vi "omni1.vi"   [LabVIEW 2012, in "Omni2013.lvrbt"]
uses:
  Omni2013.lvrbt
  <vilib>/NXT/Hardware/Plugins/Tetrix DC Motor/TetrixDCMotorAddress.ctl
  <vilib>/NXT/Hardware/Plugins/Tetrix 180 deg Servo/Tetrix180ServoAddress.ctl
  <vilib>/NXT/Dual Mode Library/Display/drawNumber_float.vi
  <vilib>/NXT/NXTIO Xnodes/NXTIONodeSubVIs/TETRIX IO Move DC Motors.vi
  <vilib>/NXT/NXTIO Xnodes/NXTIONodeSubVIs/TETRIX IO Move Servos.vi
  <vilib>/NXT/Dual Mode Library/Display/drawText_Center.vi
  <vilib>/NXT/NXTIO Xnodes/AddressXNode/NXTIOAddress.xnode
  <vilib>/NXT/NXTIO Xnodes/NXTIOXNode/NXTIO.xnode
  <vilib>/NXT/Subs/LVHSConnector.ctl
  <vilib>/NXT/LegoClasses/BrickReference/BrickReference.lvclass
panel:
  # "This VI was generated based on your configuration in the Remote Control Editor. You may modify the code as needed for your robot. To test this program for an FTC match, return to the Remote Control Editor, select the \"Run Program\" tab, and choose \"FTC Game\"."
types:
  T1 = typedef "TetrixDCMotorAddress.ctl" = i16
  T2 = cluster{"TetrixDCMotor":T1, "TetrixDCMotor 2":T1}
  T3 = typedef "LVHSConnector.ctl" = refnum<class "BrickReference.lvclass">
  T4 = typedef "FTC ControllerState.ctl" = cluster{"Left X":i8, "Left Y":i8, "Right X":i8, "Right Y":i8, "Button Encoding 9-12":u8, "Button Encoding 1-8":u8, "POV":T5}
  T5 = typedef "FTC POVState.ctl" = i8
  T6 = typedef "FTC ButtonEventType.ctl" = enum16{"Pressed", "Released"}
  T7 = cluster{"Button ID":enum16{"None", "Button 1", "Button 2", "Button 3", "Button 4", "Button 5", "Button 6", "Button 7", "Button 8", "Button 9", "Button 10", "Button 11", "Button 12", "POV Up", "POV Up Right", "POV Right", "POV Down Right", "POV Down", "POV Down Left", "POV Left", "POV Up Left"}, "Event Type":T6}[]
  T8 = enum16{"None", "Button 1", "Button 2", "Button 3", "Button 4", "Button 5", "Button 6", "Button 7", "Button 8", "Button 9", "Button 10", "Button 11", "Button 12", "POV Up", "POV Up Right", "POV Right", "POV Down Right", "POV Down", "POV Down Left", "POV Left", "POV Up Left"}
  T9 = typedef "Tetrix180ServoAddress.ctl" = i16
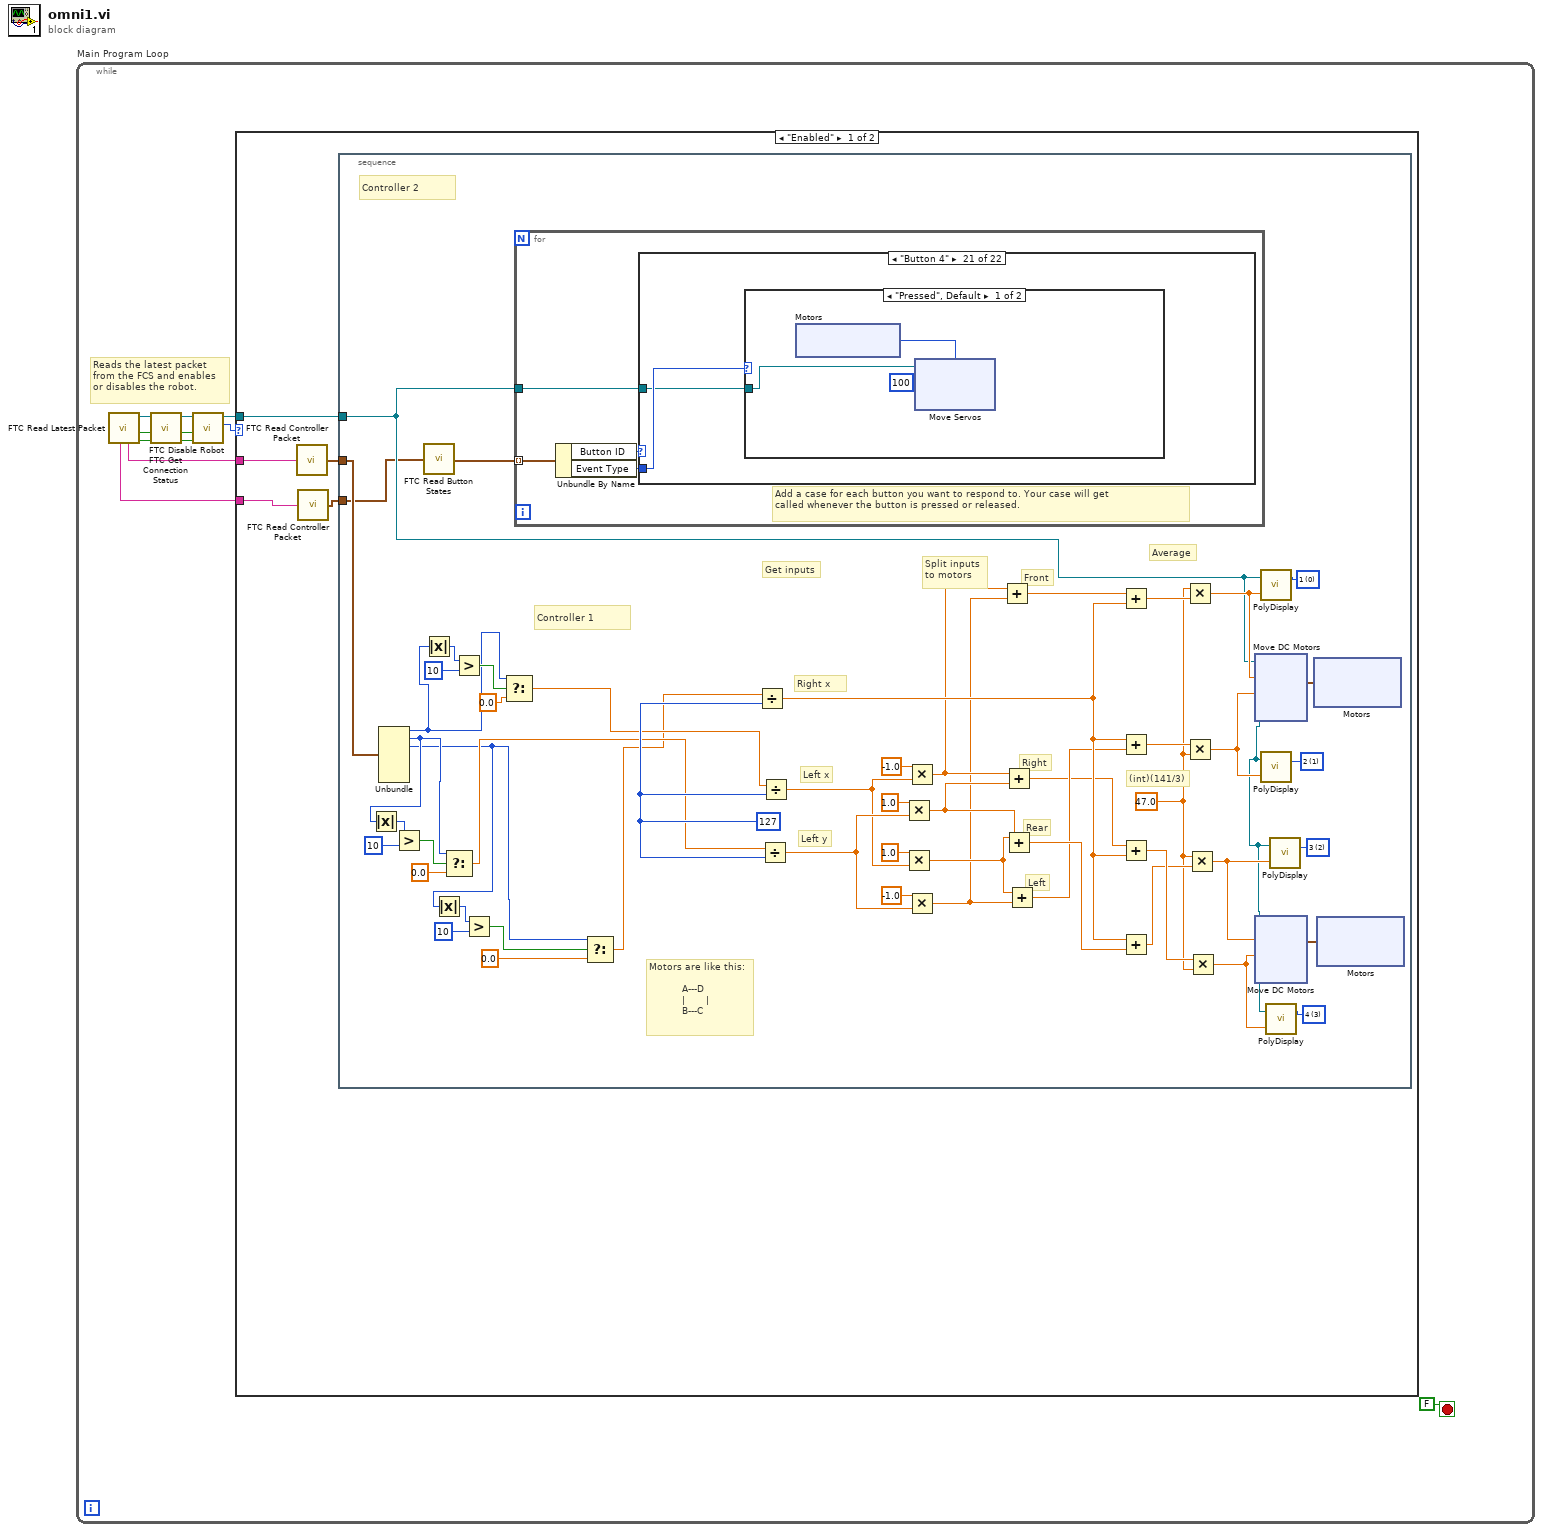
[diagram p0: block diagram]
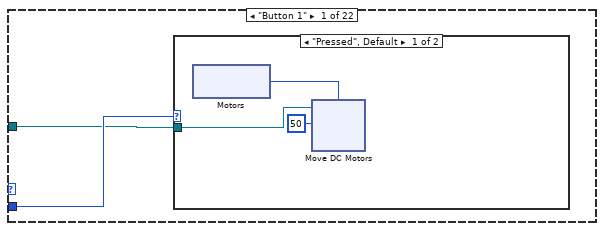
[diagram p2: hidden frame]
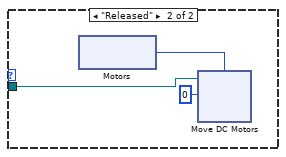
[diagram p3: hidden frame]
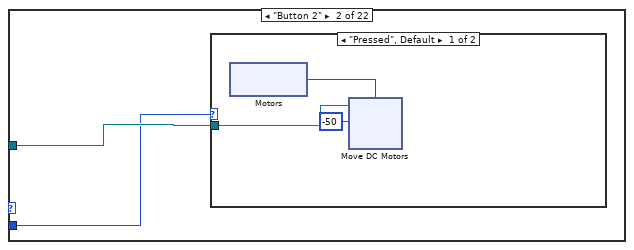
[diagram p4: hidden frame]
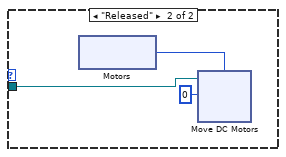
[diagram p5: hidden frame]
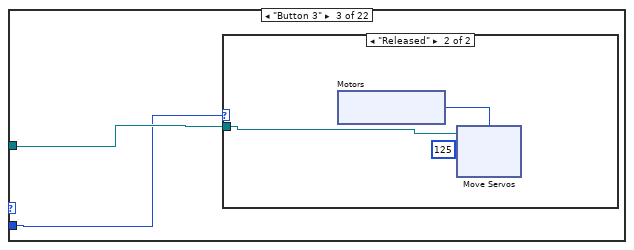
[diagram p6: hidden frame]
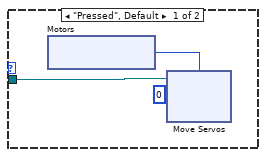
[diagram p7: hidden frame]
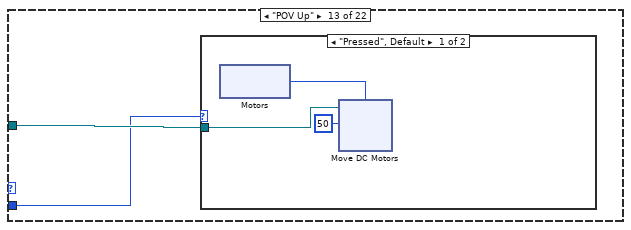
[diagram p17: hidden frame]
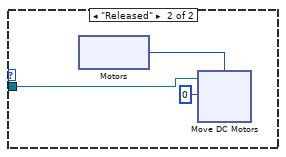
[diagram p18: hidden frame]
diagram:
  n1 = while "Main Program Loop" {
    stop <- FALSE stop-if-true
    # "Reads the latest packet\nfrom the FCS and enables\nor disables the robot."
    n2 = call <vilib>:"FTC Read Latest Packet.vi"() -> ("Packet Received?"=w9:bool, "Stopped?"=w6:bool, "NXT"=w8:T3, "Controller 1"=w10:string, "Controller 2"=w1:string)  [unwired: 6 in, 1 out]
    n3 = call <vilib>:"FTC Get Connection Status.vi"("Packet Received?"=w9, "Stopped?"=w6, "NXT"=w8) -> ("Online?"=w3:bool, "Stopped?"=w4:bool, "NXT"=w5:T3)  [unwired: 5 in]
    n4 = call <vilib>:"FTC Disable Robot.vi"("Online?"=w3, "Stopped?"=w4, "NXT"=w5) -> ("Enabled?"=w7:enum16{"Disabled", "Enabled"}, "NXT"=w2:T3)  [unwired: 3 in]
    n5 = case "disableCase" shown="\"Enabled\"" w7 {
      tunnel: w10 -> [w16 _]
      tunnel: w2 -> [w14 w249]
      tunnel: w1 -> [w13 _]
      frame "Enabled" {
        n6 = call <vilib>:"FTC Read Controller Packet.vi"("Packet"=w16) -> ("Controller State"=w15:T4)  [unwired: 4 in]
        n7 = call <vilib>:"FTC Read Controller Packet.vi"("Packet"=w13) -> ("Controller State"=w12:T4)  [unwired: 4 in]
        n8 = stacked-sequence "controller1Actions" {
          tunnel: w15 -> [w53]
          tunnel: w14 -> [w19]
          tunnel: w12 -> [w17]
          frame #0 {
            w45 = i8 127 ("y")
            w69 = i16 0 items=["1", "2", "3", "4", "5", "6", "7", "8"] ("Line")
            w68 = i16 3 items=["1", "2", "3", "4", "5", "6", "7", "8"] ("Line")
            w48 = i16 2 items=["1", "2", "3", "4", "5", "6", "7", "8"] ("Line")
            w67 = i16 1 items=["1", "2", "3", "4", "5", "6", "7", "8"] ("Line")
            w38 = 47.0 ("y")
            # "Controller 1"
            # "Average"
            # "Left"
            # "Rear"
            # "Right"
            # "Front"
            # "Motors are like this:\n\n           A---D\n           |       |\n           B---C"
            # "(int)(141/3)"
            # "Split inputs to motors"
            # "Get inputs"
            # "Left y"
            # "Right x"
            # "Left x"
            # "Controller 2"
            n9 = Unbundle(w53) -> ("Left X"=w24:i8, "Left Y"=w22:i8, "Right X"=w20:i8)  [unwired: 4 out]
            n10 = Absolute Value(x=w22) -> (abs(x)=w23:i8)
            n11 = Greater?(x=w23, y=i8 10) -> (0:w32:bool)
            n12 = call <vilib>:"FTC Read Button States.vi"("Controller State"=w17) -> ("Button Events"=w18:T7)  [unwired: 2 in, 1 out]
            n13 = Absolute Value(x=w24) -> (abs(x)=w25:i8)
            n14 = Absolute Value(x=w20) -> (abs(x)=w21:i8)
            n15 = Select(t=w22, s=w32, f=0.0) -> (s? t:f=w27:dbl)
            n16 = Greater?(x=w25, y=i8 10) -> (0:w35:bool)
            n17 = Greater?(x=w21, y=i8 10) -> (0:w29:bool)
            n18 = Select(t=w24, s=w35, f=0.0) -> (s? t:f=w28:dbl)
            n19 = for "buttonAction" {
              tunnel: w18 -> [w93] mode=indexing
              tunnel: w19 -> [w92]
              # "Add a case for each button you want to respond to. Your case will get \ncalled whenever the button is pressed or released."
              n20 = Unbundle By Name(w93) -> ("Button ID"=w95:T8, "Event Type"=w94:T6)
              n21 = case "EventCase1" shown="\"Button 4\"" w95 {
                tunnel: w94 -> [w97 w120 w144 _ _ _ _ _ _ _ _ _ w168 _ _ _ w192 _ _ _ w217 _]
                tunnel: w92 -> [w96 w121 w145 _ _ _ _ _ _ _ _ _ w169 _ _ _ w193 _ _ _ w216 _]
                frame "Button 1" {
                  n22 = case shown="\"Pressed\", Default" w97 {
                    tunnel: w96 -> [w99 w110]
                    frame "Pressed", Default {
                      n23 = xnode "Motors"() -> ("Motor"=w98:T1)
                      n24 = xnode "Move DC Motors"("Power/Speed 1"=i8 50, "Motors"=w98, "NXT"=w99) -> ()  [unwired: 1 out]
                    }
                    frame "Released" {
                      n25 = xnode "Motors"() -> ("Motor"=w109:T1)
                      n26 = xnode "Move DC Motors"("Power/Speed 1"=i8 0, "Motors"=w109, "NXT"=w110) -> ()  [unwired: 1 out]
                    }
                  }
                }
                frame "Button 2" {
                  n27 = case shown="\"Pressed\", Default" w120 {
                    tunnel: w121 -> [w123 w134]
                    frame "Pressed", Default {
                      n28 = xnode "Motors"() -> ("Motor"=w122:T1)
                      n29 = xnode "Move DC Motors"("Power/Speed 1"=i8 -50, "Motors"=w122, "NXT"=w123) -> ()  [unwired: 1 out]
                    }
                    frame "Released" {
                      n30 = xnode "Motors"() -> ("Motor"=w133:T1)
                      n31 = xnode "Move DC Motors"("Power/Speed 1"=i8 0, "Motors"=w133, "NXT"=w134) -> ()  [unwired: 1 out]
                    }
                  }
                }
                frame "Button 3" {
                  n32 = case shown="\"Released\"" w144 {
                    tunnel: w145 -> [w148 w157]
                    frame "Pressed", Default {
                      n33 = xnode "Motors"() -> ("Motor"=w146:T9)
                      n34 = xnode "Move Servos"("Position 1"=u8 0, "Servos"=w146, "NXT"=w148) -> ()  [unwired: 1 out]
                    }
                    frame "Released" {
                      n35 = xnode "Motors"() -> ("Motor"=w158:T9)
                      n36 = xnode "Move Servos"("Position 1"=u8 125, "Servos"=w158, "NXT"=w157) -> ()  [unwired: 1 out]
                    }
                  }
                }
                frame Default {
                  # "No Action"
                }
                frame "Button 5" {
                }
                frame "Button 6" {
                }
                frame "Button 7" {
                }
                frame "Button 8" {
                }
                frame "Button 9" {
                }
                frame "Button 10" {
                }
                frame "Button 11" {
                }
                frame "Button 12" {
                }
                frame "POV Up" {
                  n37 = case shown="\"Pressed\", Default" w168 {
                    tunnel: w169 -> [w171 w182]
                    frame "Pressed", Default {
                      n38 = xnode "Motors"() -> ("Motor"=w170:T1)
                      n39 = xnode "Move DC Motors"("Power/Speed 1"=i8 50, "Motors"=w170, "NXT"=w171) -> ()  [unwired: 1 out]
                    }
                    frame "Released" {
                      n40 = xnode "Motors"() -> ("Motor"=w181:T1)
                      n41 = xnode "Move DC Motors"("Power/Speed 1"=i8 0, "Motors"=w181, "NXT"=w182) -> ()  [unwired: 1 out]
                    }
                  }
                }
                frame "POV Up Right" {
                }
                frame "POV Right" {
                }
                frame "POV Down Right" {
                }
                frame "POV Down" {
                  n42 = case shown="\"Pressed\", Default" w192 {
                    tunnel: w193 -> [w195 w206]
                    frame "Pressed", Default {
                      n43 = xnode "Motors"() -> ("Motor"=w194:T1)
                      n44 = xnode "Move DC Motors"("Power/Speed 1"=i8 -50, "Motors"=w194, "NXT"=w195) -> ()  [unwired: 1 out]
                    }
                    frame "Released" {
                      n45 = xnode "Motors"() -> ("Motor"=w205:T1)
                      n46 = xnode "Move DC Motors"("Power/Speed 1"=i8 0, "Motors"=w205, "NXT"=w206) -> ()  [unwired: 1 out]
                    }
                  }
                }
                frame "POV Down Left" {
                }
                frame "POV Left" {
                }
                frame "POV Up Left" {
                }
                frame "Button 4" {
                  n47 = case shown="\"Pressed\", Default" w217 {
                    tunnel: w216 -> [w219 w230]
                    frame "Pressed", Default {
                      n48 = xnode "Motors"() -> ("Motor"=w220:T9)
                      n49 = xnode "Move Servos"("Position 1"=u8 100, "Servos"=w220, "NXT"=w219) -> ()  [unwired: 1 out]
                    }
                    frame "Released" {
                      n50 = xnode "Motors"() -> ("Motor"=w231:T9)
                      n51 = xnode "Move Servos"("Position 1"=u8 225, "Servos"=w231, "NXT"=w230) -> ()  [unwired: 1 out]
                    }
                  }
                }
                frame "None" {
                }
              }
            }
            n52 = Select(t=w20, s=w29, f=0.0) -> (s? t:f=w26:dbl)
            n53 = Divide(x=w26, y=w45) -> (x/y=w65:dbl)
            n54 = Divide(x=w27, y=w45) -> (x/y=w59:dbl)
            n55 = Divide(x=w28, y=w45) -> (x/y=w56:dbl)
            n56 = Multiply(x=1.0, y=w59) -> (x*y=w44:dbl)
            n57 = Multiply(x=1.0, y=w56) -> (x*y=w60:dbl)
            n58 = Multiply(x=-1.0, y=w56) -> (x*y=w61:dbl)
            n59 = Multiply(x=-1.0, y=w59) -> (x*y=w43:dbl)
            n60 = Add(x=w61, y=w43) -> (x+y=w64:dbl)
            n61 = Add(x=w61, y=w44) -> (x+y=w62:dbl)
            n62 = Add(x=w60, y=w44) -> (x+y=w66:dbl)
            n63 = Add(x=w60, y=w43) -> (x+y=w63:dbl)
            n64 = Add(x=w64, y=w65) -> (x+y=w40:dbl)
            n65 = Add(x=w65, y=w63) -> (x+y=w41:dbl)
            n66 = Add(x=w62, y=w65) -> (x+y=w42:dbl)
            n67 = Add(x=w65, y=w66) -> (x+y=w39:dbl)
            n68 = Multiply(x=w38, y=w40) -> (x*y=w51:dbl)
            n69 = Multiply(x=w41, y=w38) -> (x*y=w50:dbl)
            n70 = Multiply(x=w38, y=w39) -> (x*y=w46:dbl)
            n71 = Multiply(x=w42, y=w38) -> (x*y=w47:dbl)
            n72 = call-poly <vilib>:"PolyDisplay.vi"("number"=w51, "NXT"=w19, "Line"=w69) -> ()  [unwired: 1 in, 1 out]
            n73 = call-poly <vilib>:"PolyDisplay.vi"("number"=w50, "NXT"=w19, "Line"=w67) -> ()  [unwired: 1 in, 1 out]
            n74 = call-poly <vilib>:"PolyDisplay.vi"("number"=w47, "NXT"=w19, "Line"=w68) -> ()  [unwired: 1 in, 1 out]
            n75 = call-poly <vilib>:"PolyDisplay.vi"("number"=w46, "NXT"=w19, "Line"=w48) -> ()  [unwired: 1 in, 1 out]
            n76 = xnode "Motors"() -> ("Motor"=w52:cluster{"TetrixDCMotor":T1, "TetrixDCMotor":T1})
            n77 = xnode "Move DC Motors"("Power/Speed 2"=w50, "Power/Speed 1"=w51, "Motors"=w52, "NXT"=w19) -> ()  [unwired: 1 out]
            n78 = xnode "Motors"() -> ("Motor"=w49:cluster{"TetrixDCMotor":T1, "TetrixDCMotor":T1})
            n79 = xnode "Move DC Motors"("Power/Speed 2"=w47, "Power/Speed 1"=w46, "Motors"=w49, "NXT"=w19) -> ()  [unwired: 1 out]
          }
        }
      }
      frame "Disabled" {
        w242 = i16 3 items=["1", "2", "3", "4", "5", "6", "7", "8"] ("Line")
        w248 = i16 2 items=["1", "2", "3", "4", "5", "6", "7", "8"] ("Line")
        w244 = i16 1 items=["1", "2", "3", "4", "5", "6", "7", "8"] ("Line")
        n80 = call <vilib>:"FTC Display Connection Status.vi"("NXT"=w249) -> ("NXT"=w243:T3)  [unwired: 10 in]
        n81 = call-poly <vilib>:"PolyDisplay.vi"("Text"="No, You may not ", "NXT"=w243, "Line"=w244) -> ("NXT"=w246:T3)  [unwired: 1 in]
        n82 = call-poly <vilib>:"PolyDisplay.vi"("Text"="connect. I am ", "NXT"=w246, "Line"=w248) -> ("NXT"=w241:T3)  [unwired: 1 in]
        n83 = call-poly <vilib>:"PolyDisplay.vi"("Text"="mad at you.", "NXT"=w241, "Line"=w242) -> ()  [unwired: 1 in, 1 out]
      }
    }
  }
